vi "Write Target Name.vi"(8 "error in (no error)":errorcluster, 10 "Target Name":string="myRIO Target", 11 "myRIOMetaDataObj in":refnum<class "myRIOMetaDataObj.lvclass">) -> (0 "error out":errorcluster, 3 "myRIOMetaDataObj out":refnum<class "myRIOMetaDataObj.lvclass">)   [LabVIEW 2021, in "myRIOMetaDataObj.lvclass"]
uses:
  myRIOMetaDataObj.lvclass
  myRIOMetaDataObj.lvclass/myRIOMetaDataObj.ctl
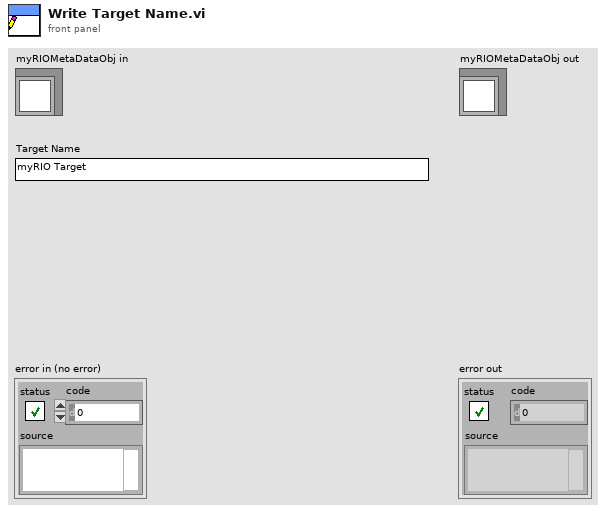
[diagram p1: front panel]
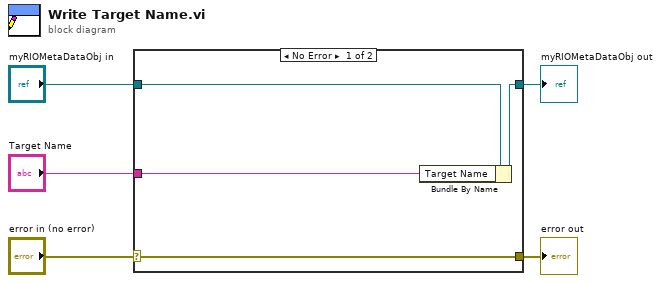
[diagram p0: block diagram]
diagram:
  n1 = case shown="No Error" "error in (no error)" {
    selector: "error in (no error)" -> [w9 w10]
    tunnel: [w9 w10] -> w4
    tunnel: [w7 w11] -> w2
    tunnel: "myRIOMetaDataObj in" -> [w8 w11]
    tunnel: "Target Name" -> [w6 _]
    frame No Error {
      n2 = Bundle By Name(cluster=w8, "Target Name"=w6) -> (w7:refnum<class "myRIOMetaDataObj.lvclass">)
    }
    frame Error {
    }
  }
  "error out" <- w4
  "myRIOMetaDataObj out" <- w2
